vi "factorial using for loop.vi"() -> ()   [LabVIEW 2018]
panel:
  out "Loop Count":i32
  out "result":u32
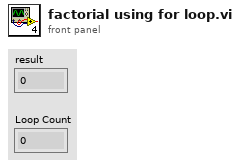
[diagram p1: front panel]
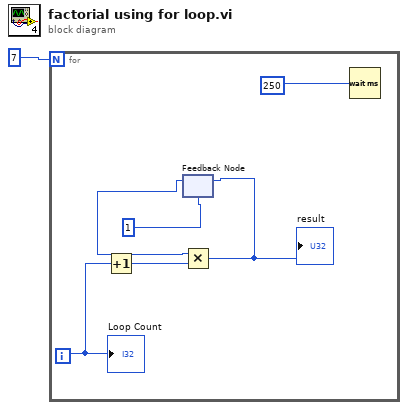
[diagram p0: block diagram]
diagram:
  n1 = for {
    N: 7 -> [_]
    i -> [w3]
    n2 = Increment(x=w3) -> (x+1=w2:i32)
    n3 = feedback #1(u8 1) -> (w4:u8)
    n4 = Multiply(x=w4, y=w2) -> (x*y=w5:i32)
    "result" <- w5
    n5 = feedback-in #1(w5) -> ()
    n6 = Wait (ms)(milliseconds to wait=u32 250) -> ()  [unwired: 1 out]
    "Loop Count" <- w3
  }
